vi "GUI.vi"(8 "error in":errorcluster, 11 "SequenceContext":refnum<k7>) -> (0 "error out":errorcluster)   [LabVIEW 2021, in "User Console.lvlib"]
uses:
  User Console.lvlib
  Controls/Images.ctl
  <vilib>/addons/TestStand/_TSUtility.llb/TestStand - Start Modal Dialog (Sequence Context).vi
  <vilib>/addons/TestStand/_TSUtility.llb/TestStand - End Modal Dialog (Sequence Context).vi
panel:
  in  "FileNames":T1 items=["DMM Expand.jpg", "ACIR Expand.jpg", "DMM Retract.jpg", "ACIR Retract.jpg", "Retract All.jpg"]
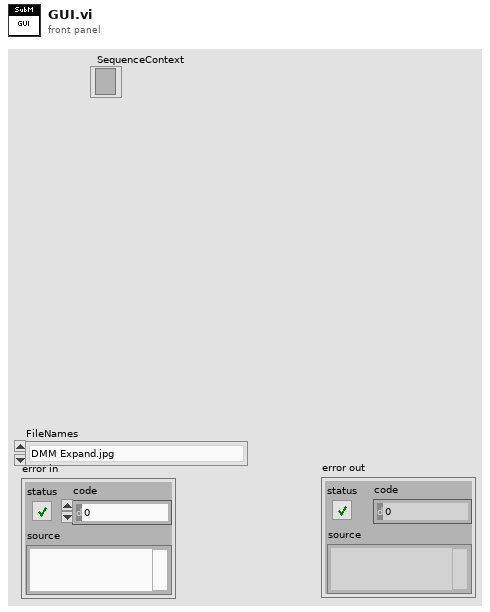
[diagram p1: front panel]
types:
  T1 = typedef "Images.ctl" = u16
  T2 = typedef "imagedata.ctl" = cluster{"image type":i32, "image depth":i32, "image":u8[], "mask":u8[], "colors":u32[], "Rectangle":cluster{"left":i16, "top":i16, "right":i16, "bottom":i16}}
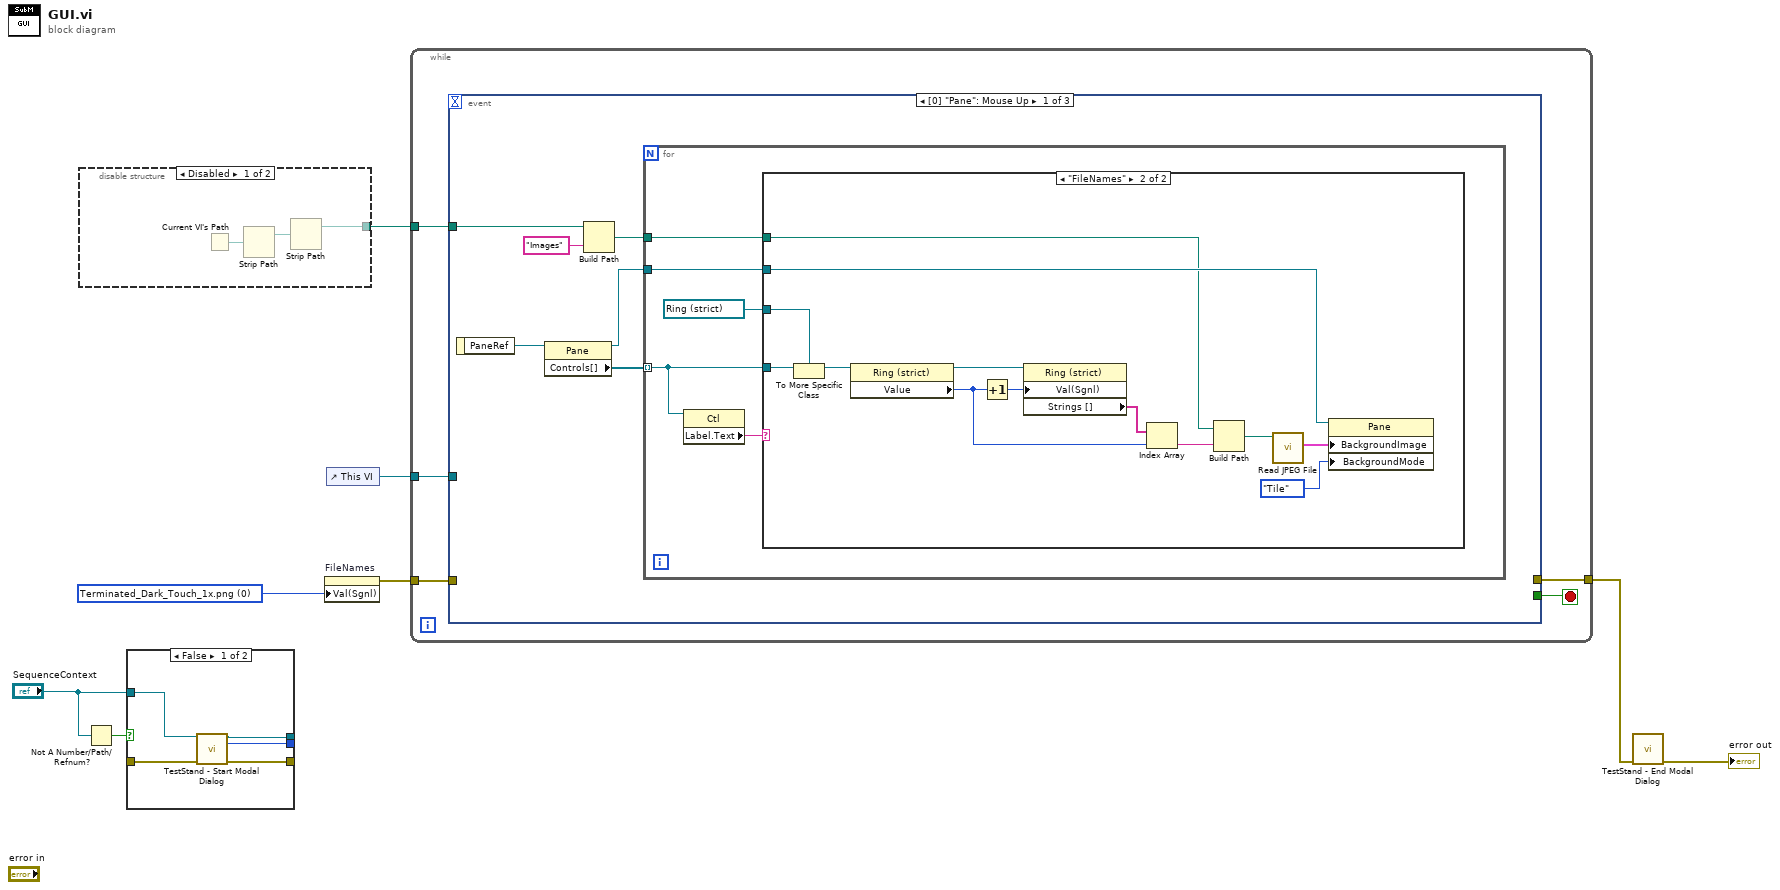
[diagram p0: block diagram]
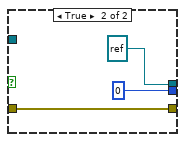
[diagram p2: hidden frame]
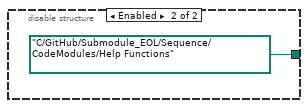
[diagram p3: hidden frame]
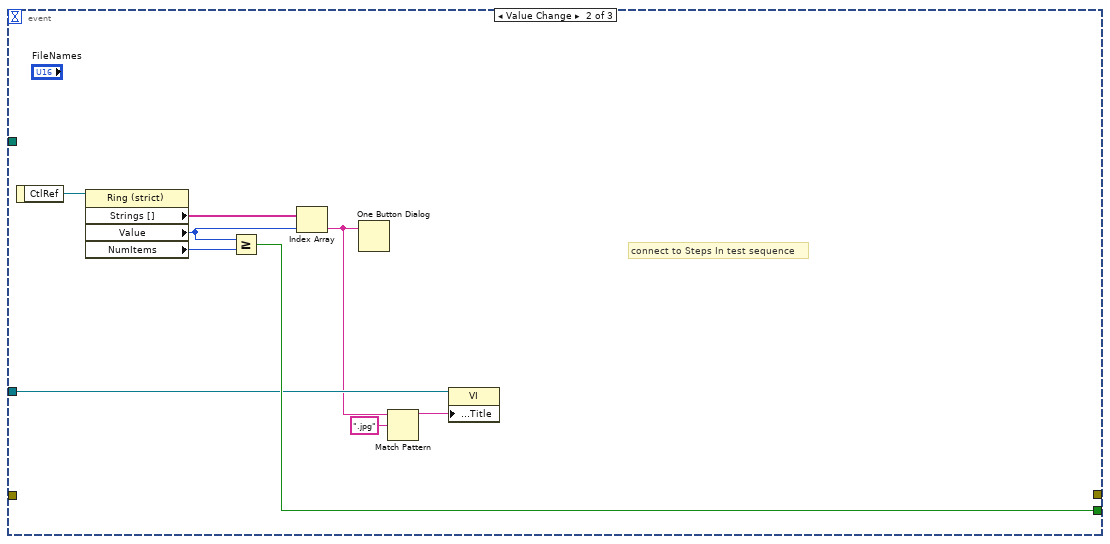
[diagram p5: hidden frame]
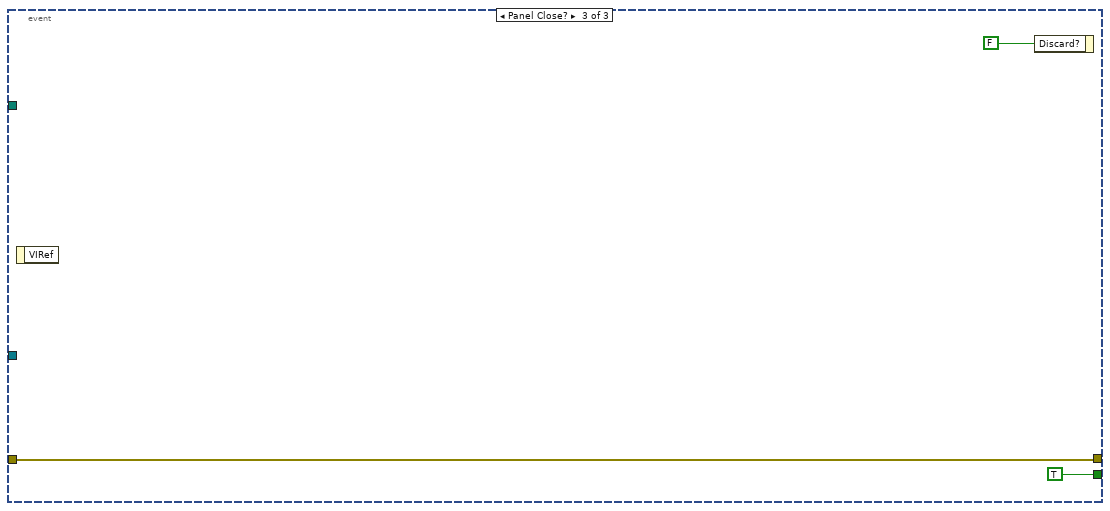
[diagram p6: hidden frame]
diagram:
  w7 = T1 0 items=["Terminated_Dark_Touch_1x.png", "Pass_Dark_Touch_1x.png", "Fail_Dark_Touch_1x.png", "Error_Dark_Touch_1x.png"] ("FileNames")
  n1 = disable-structure shown="Disabled" {
    disable-tunnel: [w9 path "C:/GitHub/Submodule_EOL/Sequence/CodeModules/Help Functions" ("stripped path")] -> w6
    frame Disabled {
      n2 = Current VI's Path() -> (path=w11:path)
      n3 = Strip Path(path=w11) -> (stripped path=w10:path)  [unwired: 1 out]
      n4 = Strip Path(path=w10) -> (stripped path=w9:path)  [unwired: 1 out]
    }
    frame Enabled {
    }
  }
  n5 = Not A Number/Path/Refnum?(number/path/refnum="SequenceContext") -> (NaN/Path/Refnum?=w3:bool)
  n6 = case shown="False" w3 {
    tunnel: _ -> [w16 w20]
    tunnel: [w15 w20] -> _
    tunnel: "SequenceContext" -> [w17 _]
    tunnel: [w14 refnum<k7> refnum ("Sequence Context Out")] -> _
    tunnel: [w13 0 ("Modal ID")] -> _
    frame False {
      n7 = call-poly <vilib>:"TestStand - Start Modal Dialog.vi"("Sequence Context In"=w17, "error in (no error)"=w16) -> ("Sequence Context Out"=w14:refnum<k7>, "Modal ID"=w13:i32, "error out"=w15:errorcluster)  [unwired: 9 in, 2 out]
    }
    frame True {
    }
  }
  n8 = property on="FileNames" class="Ring (strict)"("Val(Sgnl)"=w7) -> (error out=w8:errorcluster)  [unwired: 2 in, 1 out]
  n9 = control-ref of="This VI"() -> (w5:refnum<vi>)
  n10 = while {
    tunnel: w8 -> [w24]
    tunnel: [w23] -> w1
    tunnel: w6 -> [w22]
    tunnel: w5 -> [w21]
    stop <- w25 stop-if-true
    n11 = event shown="[0] \"Pane\": Mouse Up" {
      selector: _ -> [_ _ _]
      dyn-events: _ -> [_ _ _]
      timeout: _ -> [_ _ _]
      tunnel: [_ w56 TRUE ("Discard?")] -> w25
      tunnel: w24 -> [_ _ w59]
      tunnel: [_ _ w59] -> w23
      tunnel: w22 -> [w27 _ _]
      tunnel: w21 -> [_ w53 _]
      event Mouse Up {
        n12 = event-data() -> ("PaneRef"=w30:refnum<vi>)  [unwired: 1 in]
        n13 = property class="Pane"(reference=w30) -> (reference out=w29:refnum<vi>, "Controls[]"=w31:refnum<vi>[])  [unwired: 1 in, 1 out]
        n14 = Build Path(base path=w27, name or relative path="Images") -> (appended path=w26:path)
        n15 = for {
          tunnel: w31 -> [w35] mode=indexing
          tunnel: w29 -> [w33]
          tunnel: w26 -> [w32]
          n16 = property class="Ctl"(reference=w35) -> ("Label.Text"=w36:string)  [unwired: 1 in, 2 out]
          n17 = case shown="\"FileNames\"" w36 {
            tunnel: w35 -> [_ w46]
            tunnel: refnum<vi> refnum ("FileNames") -> [_ w45]
            tunnel: w33 -> [_ w38]
            tunnel: w32 -> [_ w37]
            frame Default {
            }
            frame "FileNames" {
              n18 = To More Specific Class(target class=w45, reference=w46) -> (specific class reference=w43:refnum<vi>)  [unwired: 1 in, 1 out]
              n19 = property class="Ring (strict)"(reference=w43) -> (reference out=w41:refnum<vi>, "Value"=w39:T1)  [unwired: 1 in, 1 out]
              n20 = Increment(x=w39) -> (x+1=w44:T1)
              n21 = property class="Ring (strict)"(reference=w41, "Val(Sgnl)"=w44) -> ("Strings []"=w40:string[])  [unwired: 1 in, 2 out]
              n22 = Index Array(array=w40, index=w39) -> (element=w42:string)
              n23 = Build Path(base path=w37, name or relative path=w42) -> (appended path=w48:path)
              n24 = call <vilib>:"Read JPEG File.vi"("path to JPEG file"=w48) -> ("image data"=w49:T2)  [unwired: 8 in, 2 out]
              n25 = property class="Pane"(reference=w38, "BackgroundImage"=w49, "BackgroundMode"=enum16{"Stretch", "Center", "Tile"}."Tile" ("Background Mode")) -> ()  [unwired: 1 in, 2 out]
            }
          }
        }
      }
      event Value Change {
        # "connect to Steps In test sequence"
        n26 = event-data() -> ("CtlRef"=w58:refnum<vi>)  [unwired: 1 in]
        n27 = property class="Ring (strict)"(reference=w58) -> ("Strings []"=w55:string[], "Value"=w54:T1, "NumItems"=w57:u32)  [unwired: 1 in, 2 out]
        n28 = Greater Or Equal?(x=w54, y=w57) -> (x >= y?=w56:bool)
        n29 = Index Array(array=w55, index=w54) -> (element=w52:string)
        n30 = One Button Dialog(message=w52) -> ()  [unwired: 1 in, 1 out]
        n31 = Match Pattern(string=w52, regular expression=".jpg") -> (before substring=w50:string)  [unwired: 1 in, 3 out]
        n32 = property class="VI"(reference=w53, "Front Panel.Title"=w50) -> ()  [unwired: 1 in, 2 out]
      }
      event Panel Close? {
        n33 = event-data() -> ()  [unwired: 1 in, 1 out]
        n34 = event-data("Discard?"=FALSE) -> ()  [unwired: 1 in, 1 out]
      }
    }
  }
  n35 = call-poly <vilib>:"TestStand - End Modal Dialog.vi"("error in (no error)"=w1) -> ("error out"=→"error out":errorcluster)  [unwired: 14 in]
